vi "Read Type.vi"(8 "Error In":errorcluster, 11 "Section In":refnum<class "Section.lvclass">) -> (0 "Error Out":errorcluster, 2 "Type":T1=enum."Unknown", 3 "Section Out":refnum<class "Section.lvclass">)   [LabVIEW 2018, in "Toolkit.lvlib" / "Nodes.lvlib" / "Section.lvclass"]
doc: "Gets the Node type. LabVIEW 2009 does not have the Get LV Class Name function, so this is a workaround to determine the Node class/type during run-time."
uses:
  Section.lvclass
  Type Definitions/Types.ctl
  Nodes.lvlib
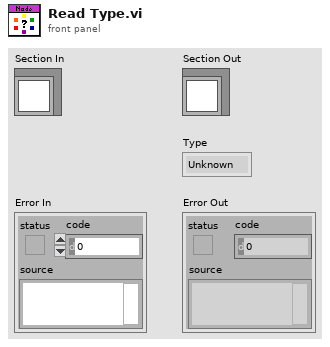
[diagram p1: front panel]
types:
  T1 = typedef "Toolkit.lvlib/Nodes.lvlib/Types.ctl" = enum16{"Comment", "Delimiter", "Partial", "Root", "Section", "Text", "Unknown", "Variable"}
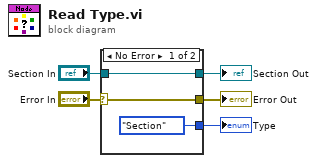
[diagram p0: block diagram]
diagram:
  n1 = case shown="No Error" "Error In" {
    selector: "Error In" -> [w8 w10]
    tunnel: [w8 w10] -> w4
    tunnel: "Section In" -> [w7 w9]
    tunnel: [w7 w9] -> w2
    tunnel: [Types."Section" ("Type") _] -> w1
    frame No Error {
    }
    frame Error {
    }
  }
  "Error Out" <- w4
  "Section Out" <- w2
  "Type" <- w1
